vi "OA_NewEmptyGraph.vi"(4 "Show":bool=TRUE, 5 "Template Name":string="origin", 6 "error in (no error)":errorcluster, 7 "Origin.IOApplication":refnum<k7>) -> (0 "error out":errorcluster, 1 "Origin.GraphLayer":refnum<k7>, 2 "Origin.GraphPage":refnum<k7>, 3 "Origin.IOApplication":refnum<k7>)   [LabVIEW 2010]
doc: "Create an empty graph window\n\nTemplate Name:\n Template file name, .otp extention is not needed.\n if no path is specified, will search Origin folders starting from the \n User Folder, the Group Folder and the Program Folder\nShow:\n Show or Hide the newly added graph window"
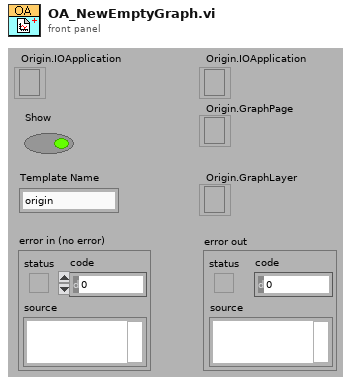
[diagram p1: front panel]
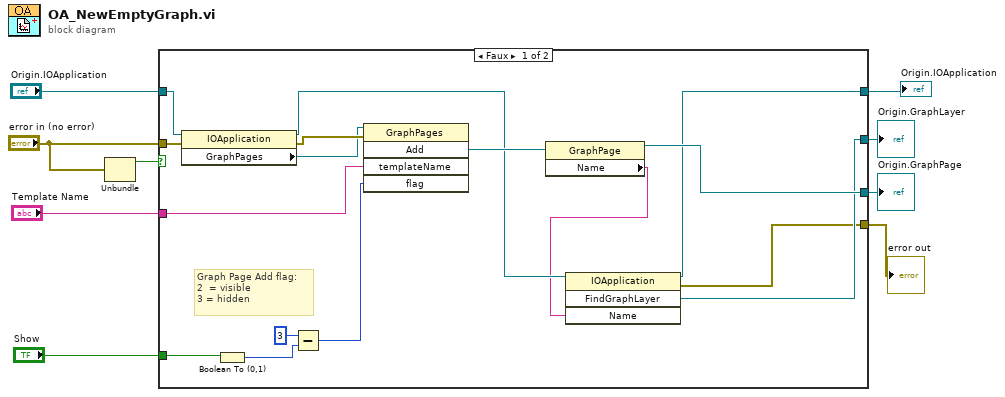
[diagram p0: block diagram]
diagram:
  n1 = Unbundle("error in (no error)") -> ("status"=w9:bool)  [unwired: 2 out]
  n2 = case shown="Faux" w9 {
    tunnel: "Origin.IOApplication" -> [w24 w27]
    tunnel: [w11 w27] -> w7
    tunnel: "error in (no error)" -> [w25 w26]
    tunnel: "Template Name" -> [w21 _]
    tunnel: "Show" -> [w23 _]
    tunnel: [w12 w26] -> w3
    tunnel: [w17 _] -> w2
    tunnel: [w13 _] -> w1
    frame False {
      # "Graph Page Add flag: \n2  = visible\n3 = hidden"
      n3 = property class="IOApplication"(reference=w24, error in=w25) -> (reference out=w15:refnum<k7>, error out=w22:errorcluster, "GraphPages"=w10:refnum<k7>)
      n4 = Boolean To (0,1)(Boolean=w23) -> (0, 1=w19:i16)
      n5 = Subtract(x=3, y=w19) -> (x-y=w18:i32)
      n6 = invoke class="GraphPages" method="Add"(reference=w10, error in=w22, "templateName"=w21, "flag"=w18) -> ("Add"=w16:refnum<k7>)  [unwired: 1 in, 4 out]
      n7 = property class="GraphPage"(reference=w16) -> (reference out=w17:refnum<k7>, "Name"=w14:string)  [unwired: 1 in, 1 out]
      n8 = invoke class="IOApplication" method="FindGraphLayer"(reference=w15, "Name"=w14) -> (reference out=w11:refnum<k7>, error out=w12:errorcluster, "FindGraphLayer"=w13:refnum<k7>)  [unwired: 2 in, 1 out]
    }
    frame True {
    }
  }
  "Origin.IOApplication" <- w7
  "error out" <- w3
  "Origin.GraphLayer" <- w1
  "Origin.GraphPage" <- w2
